vi "sendMultiple.vi"(0 "refer":refnum<queue>[](array[refnum]), 1 "to":string, 2 "from":string, 3 "data":variant, 4 "priority":bool, 5 "errorIn":errorcluster, 6 "remark1":string, 7 "Index":i32, 8 "remark 2":string) -> (14 "refer":refnum<queue>, 19 "errorOut":errorcluster)   [LabVIEW 2017]
uses:
  models/EMSGData.ctl
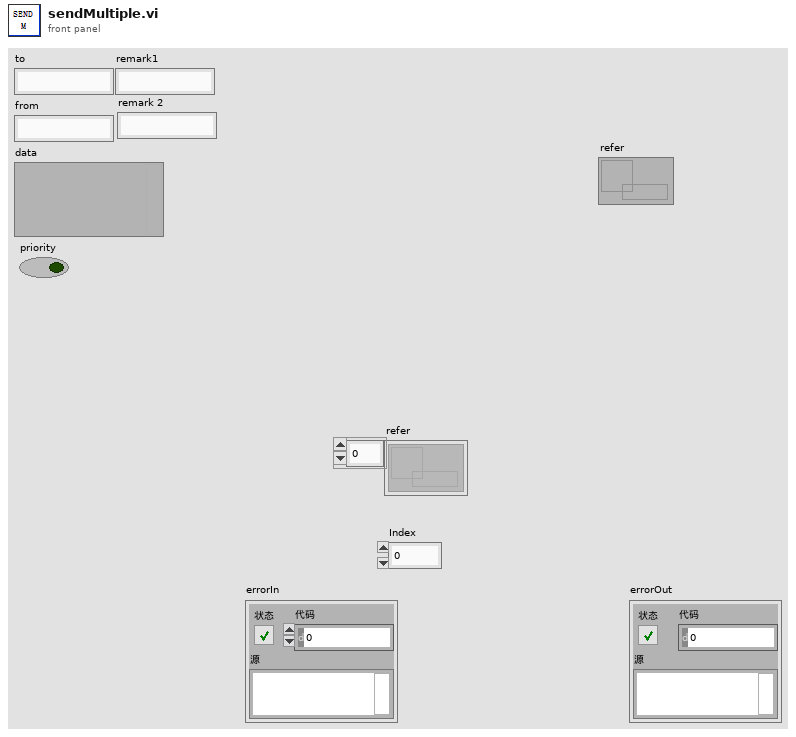
[diagram p1: front panel]
types:
  T1 = typedef "EMSGData.ctl" = cluster{"to":string, "from":string, "data":variant, "remark1":string, "remark 2":string}
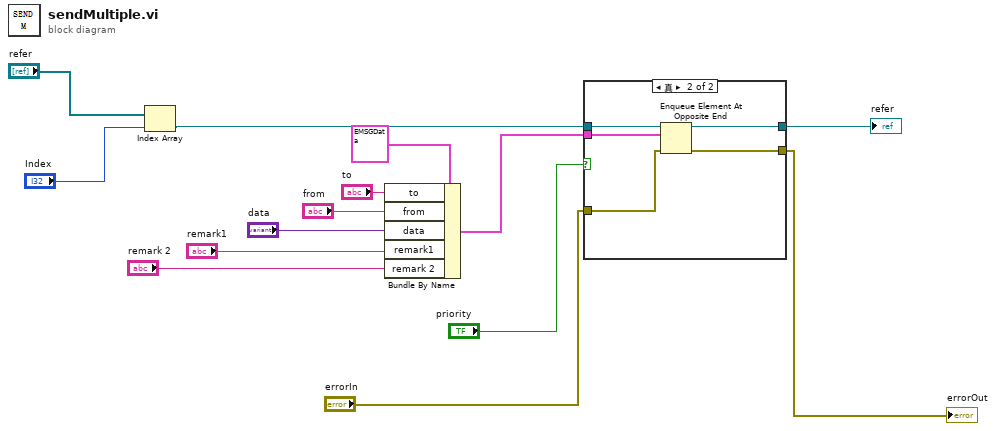
[diagram p0: block diagram]
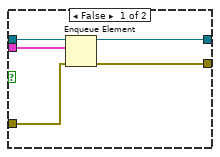
[diagram p2: hidden frame]
diagram:
  n1 = Index Array(array="refer", index="Index") -> (element=w1:refnum<queue>)
  n2 = Bundle By Name(cluster=T1 {"to"="", "from"="", "data"=variant, "remark1"="", "remark 2"=""} ("EMSGData"), "to"="to", "from"="from", "data"="data", "remark1"="remark1", "remark 2"="remark 2") -> (w8:T1)
  n3 = case shown="真" "priority" {
    tunnel: w1 -> [w19 w24]
    tunnel: w8 -> [w18 w23]
    tunnel: "errorIn" -> [w17 w22]
    tunnel: [w16 w21] -> w5
    tunnel: [w15 w20] -> w4
    frame False {
      n4 = Enqueue Element(queue=w19, element=w18, error in (no error)=w17) -> (queue out=w15:refnum<queue>, error out=w16:errorcluster)  [unwired: 1 in, 1 out]
    }
    frame True {
      n5 = Enqueue Element At Opposite End(queue=w24, element=w23, error in (no error)=w22) -> (queue out=w20:refnum<queue>, error out=w21:errorcluster)  [unwired: 1 in, 1 out]
    }
  }
  "errorOut" <- w5
  "refer" <- w4
